vi "InsertDevicePanel.vi"(0 "Communication in":refnum<class "MicroscopeController.lvclass">, 5 "Panel":string, 9 "VI Refnum":refnum<vi>, 11 "error in (no error)":errorcluster) -> (4 "Communication out":refnum<class "MicroscopeController.lvclass">, 15 "error out":errorcluster)   [LabVIEW 2020, in "MicroscopeController.lvlib" / "MicroscopeController.lvclass"]
uses:
  MicroscopeController.lvclass
  MicroscopeController.lvclass/MicroscopeController.ctl
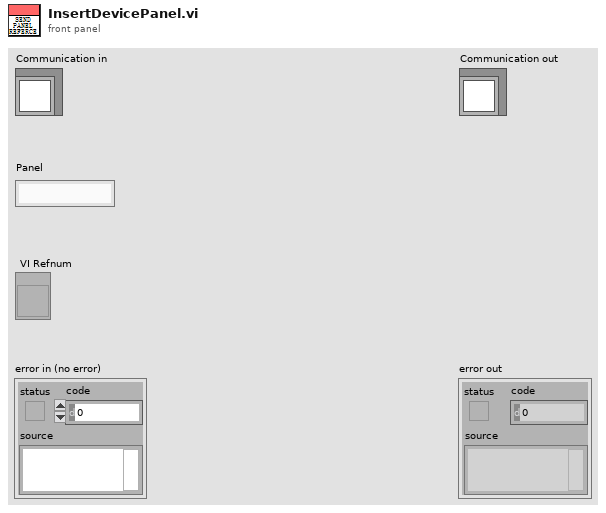
[diagram p1: front panel]
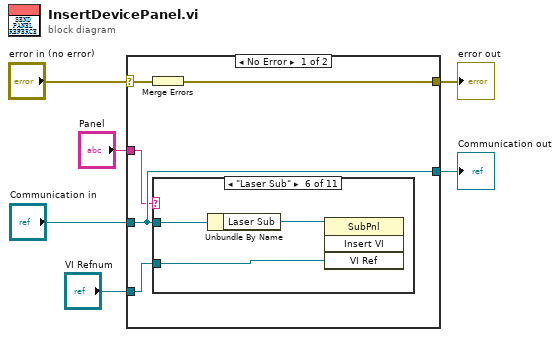
[diagram p0: block diagram]
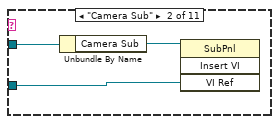
[diagram p3: hidden frame]
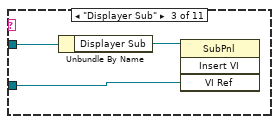
[diagram p4: hidden frame]
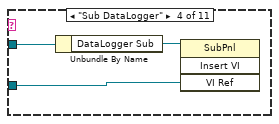
[diagram p5: hidden frame]
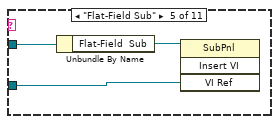
[diagram p6: hidden frame]
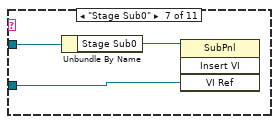
[diagram p7: hidden frame]
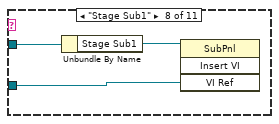
[diagram p8: hidden frame]
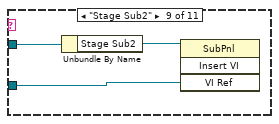
[diagram p9: hidden frame]
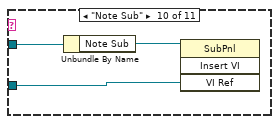
[diagram p10: hidden frame]
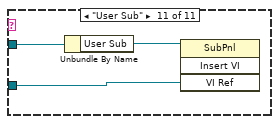
[diagram p11: hidden frame]
diagram:
  n1 = case shown="No Error" "error in (no error)" {
    selector: "error in (no error)" -> [w10 w43]
    tunnel: [w9 w43] -> w5
    tunnel: [w11 w42] -> w4
    tunnel: "Communication in" -> [w11 w42]
    tunnel: "VI Refnum" -> [w8 _]
    tunnel: "Panel" -> [w7 _]
    frame No Error {
      n2 = Merge Errors(w10) -> (w9:errorcluster)
      n3 = case shown="\"Laser Sub\"" w7 {
        tunnel: w11 -> [_ w14 w17 w20 w23 w26 w29 w32 w35 w38 w41]
        tunnel: w8 -> [_ w12 w15 w18 w21 w24 w27 w30 w33 w36 w39]
        frame Default {
        }
        frame "Camera Sub" {
          n4 = Unbundle By Name(w14) -> ("Camera Sub"=w13:refnum<vi>)
          n5 = invoke class="SubPnl" method="Insert VI"(reference=w13, "VI Ref"=w12) -> ()  [unwired: 2 in, 4 out]
        }
        frame "Displayer Sub" {
          n6 = Unbundle By Name(w17) -> ("Displayer Sub"=w16:refnum<vi>)
          n7 = invoke class="SubPnl" method="Insert VI"(reference=w16, "VI Ref"=w15) -> ()  [unwired: 2 in, 4 out]
        }
        frame "Sub DataLogger" {
          n8 = Unbundle By Name(w20) -> ("DataLogger Sub"=w19:refnum<vi>)
          n9 = invoke class="SubPnl" method="Insert VI"(reference=w19, "VI Ref"=w18) -> ()  [unwired: 2 in, 4 out]
        }
        frame "Flat-Field Sub" {
          n10 = Unbundle By Name(w23) -> ("Flat-Field  Sub"=w22:refnum<vi>)
          n11 = invoke class="SubPnl" method="Insert VI"(reference=w22, "VI Ref"=w21) -> ()  [unwired: 2 in, 4 out]
        }
        frame "Laser Sub" {
          n12 = Unbundle By Name(w26) -> ("Laser Sub"=w25:refnum<vi>)
          n13 = invoke class="SubPnl" method="Insert VI"(reference=w25, "VI Ref"=w24) -> ()  [unwired: 2 in, 4 out]
        }
        frame "Stage Sub0" {
          n14 = Unbundle By Name(w29) -> ("Stage Sub0"=w28:refnum<vi>)
          n15 = invoke class="SubPnl" method="Insert VI"(reference=w28, "VI Ref"=w27) -> ()  [unwired: 2 in, 4 out]
        }
        frame "Stage Sub1" {
          n16 = Unbundle By Name(w32) -> ("Stage Sub1"=w31:refnum<vi>)
          n17 = invoke class="SubPnl" method="Insert VI"(reference=w31, "VI Ref"=w30) -> ()  [unwired: 2 in, 4 out]
        }
        frame "Stage Sub2" {
          n18 = Unbundle By Name(w35) -> ("Stage Sub2"=w34:refnum<vi>)
          n19 = invoke class="SubPnl" method="Insert VI"(reference=w34, "VI Ref"=w33) -> ()  [unwired: 2 in, 4 out]
        }
        frame "Note Sub" {
          n20 = Unbundle By Name(w38) -> ("Note Sub"=w37:refnum<vi>)
          n21 = invoke class="SubPnl" method="Insert VI"(reference=w37, "VI Ref"=w36) -> ()  [unwired: 2 in, 4 out]
        }
        frame "User Sub" {
          n22 = Unbundle By Name(w41) -> ("User Sub"=w40:refnum<vi>)
          n23 = invoke class="SubPnl" method="Insert VI"(reference=w40, "VI Ref"=w39) -> ()  [unwired: 2 in, 4 out]
        }
      }
    }
    frame Error {
    }
  }
  "error out" <- w5
  "Communication out" <- w4
